vi "Recibir datos.vi"() -> ()   [LabVIEW 2020]
uses:
  <vilib>/httpClient/LabVIEWHTTPClient.lvlib
panel:
  out "body GET":string
  out "headers GET":string
  out "Acondicionamiento":dbl
  out "Data":string
  out "Hora":string
  out "Led rele":bool
  in  "stop":bool
  out "error GET":errorcluster
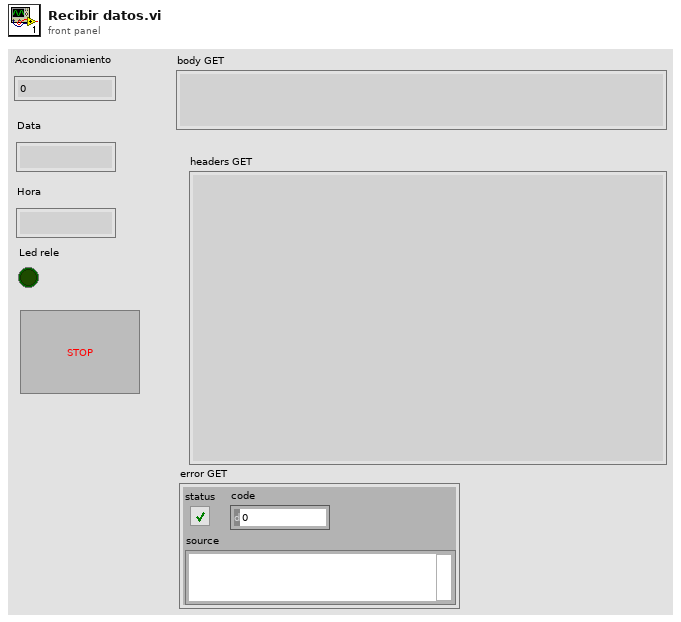
[diagram p1: front panel]
types:
  T1 = cluster{"Acondicionamiento":dbl, "Data":string, "Hora":string, "Led rele":bool}
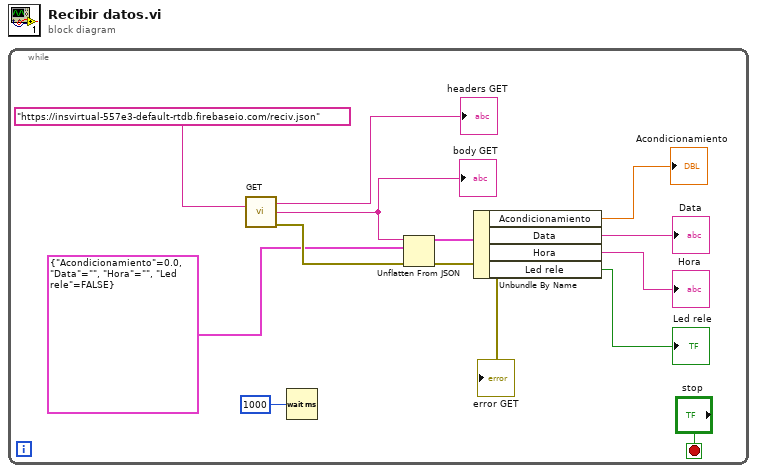
[diagram p0: block diagram]
diagram:
  n1 = while {
    stop <- "stop" stop-if-true
    n2 = call <vilib>:"GET.vi"("url"="https://insvirtual-557e3-default-rtdb.firebaseio.com/reciv.json") -> ("headers"=→"headers GET":string, "body"=w3:string, "error out"=w4:errorcluster)  [unwired: 11 in, 1 out]
    "body GET" <- w3
    n3 = Wait (ms)(milliseconds to wait=u32 1000) -> ()  [unwired: 1 out]
    n4 = Unflatten From JSON(JSON string=w3, type and defaults=T1 {"Acondicionamiento"=0.0, "Data"="", "Hora"="", "Led rele"=FALSE}, error in (no error)=w4) -> (value=w2:T1, error out=→"error GET":errorcluster)  [unwired: 4 in]
    n5 = Unbundle By Name(w2) -> ("Acondicionamiento"=→"Acondicionamiento":dbl, "Data"=→"Data":string, "Hora"=→"Hora":string, "Led rele"=→"Led rele":bool)
  }
